vi "GraphsUpdateRaw.vi"(10 "data in":i32[][](array[numeric]), 11 "GraphChart in":refnum<vi>) -> ()   [LabVIEW 2019]
panel:
  out "Waveform Graph":i32[][](graph)
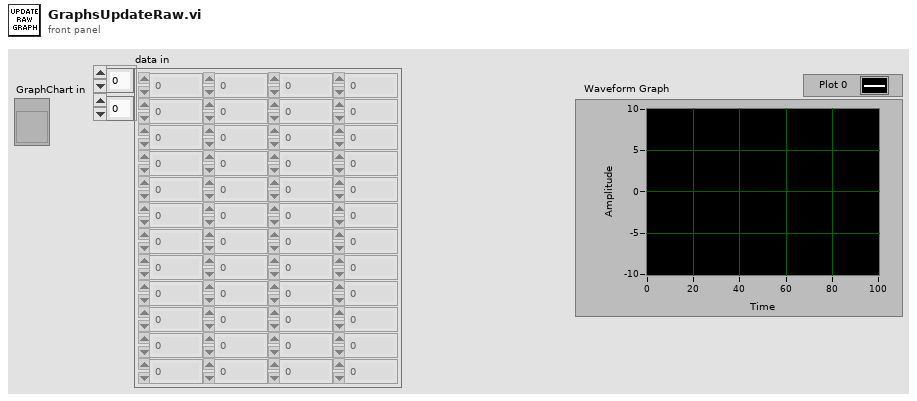
[diagram p1: front panel]
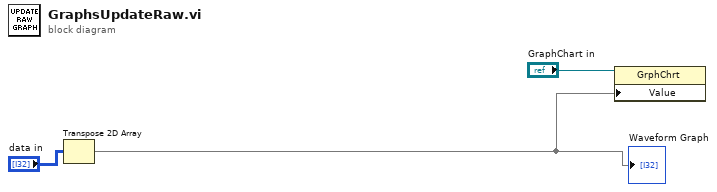
[diagram p0: block diagram]
diagram:
  n1 = Transpose 2D Array(2D array="data in") -> (transposed array=w1:i32[][])
  "Waveform Graph" <- w1
  n2 = property class="GrphChrt"(reference="GraphChart in", "Value"=w1) -> ()  [unwired: 1 in, 2 out]
